vi "AddToArraySmall.vi"(11 "Input":dbl) -> (3 "output array":dbl[](array[numeric]))   [LabVIEW 2022 SP3]
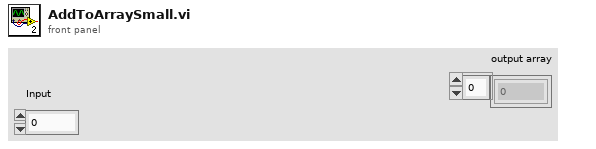
[diagram p1: front panel]
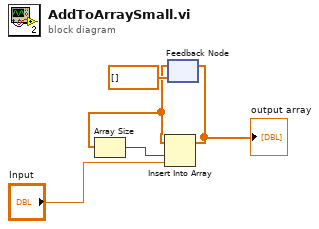
[diagram p0: block diagram]
diagram:
  n1 = feedback #1(dbl[] []) -> (w1:dbl[])
  n2 = Array Size(array=w1) -> (size(s)=w2:i32)
  n3 = Insert Into Array(array=w1, index=w2, new element="Input") -> (w4:dbl[])
  "output array" <- w4
  n4 = feedback-in #1(w4) -> ()
